vi "Temperature Conversion.vi"(11 "Temperature F":dbl(knob)=32.0 scale=0.0..100.0) -> (3 "Temperature C":dbl)   [LabVIEW 2014]
panel:
  out "String":string
  in  "Stop":bool
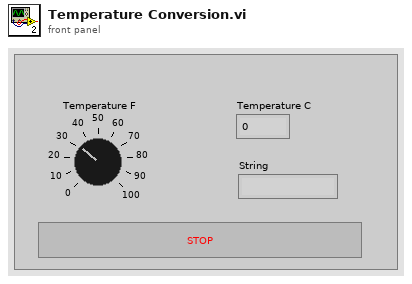
[diagram p1: front panel]
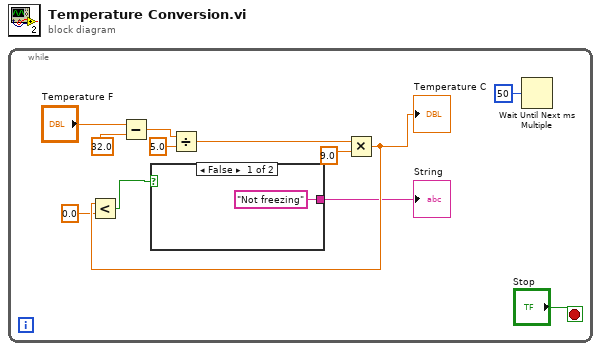
[diagram p0: block diagram]
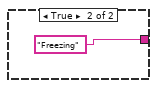
[diagram p2: hidden frame]
diagram:
  n1 = while {
    stop <- "Stop" stop-if-true
    n2 = Subtract(x="Temperature F", y=32.0) -> (x-y=w10:dbl)
    n3 = Divide(x=w10, y=5.0) -> (x/y=w8:dbl)
    n4 = Multiply(x=w8, y=9.0) -> (x*y=w4:dbl)
    "Temperature C" <- w4
    n5 = Less?(x=w4, y=0.0) -> (x < y?=w2:bool)
    n6 = case shown="False" w2 {
      tunnel: ["Not freezing" ("String") "Freezing" ("String")] -> w1
      frame False {
      }
      frame True {
      }
    }
    "String" <- w1
    n7 = Wait Until Next ms Multiple(millisecond multiple=u32 50) -> ()  [unwired: 1 out]
  }
